vi "DB - OFFSET FETCH.vi"(5 "Include Inactive":bool=TRUE, 6 "OFFSET ROW":i32, 7 "subVI":bool=TRUE, 8 "error in (no error)":errorcluster, 9 "Column to Order BY":string="orderid", 10 "DB.dbo.Table":string="MyDB1.dbo.PartsDetails", 11 "Refnum in":T3) -> (0 "error out":errorcluster, 2 "Data":string[](array[string]), 3 "Refnum out":T3)   [LabVIEW 2013]
uses:
  <vilib>/addons/database/Connection.llb/Conn ObjectReference.ctl
  Controls/DB - DB.Schema.Table.ctl
  <vilib>/addons/database/Connection.llb/Conn Execute.vi
  <vilib>/addons/database/Recordset.llb/Rec Fetch Recordset Data (R).vi
  <vilib>/addons/database/Recordset.llb/Rec Destroy - Connection.vi
  <vilib>/addons/database/Connection.llb/DB Tools Open Connec (String).vi
  <vilib>/addons/database/_DB Variant To Data/Database Variant To Data.xnode
  <vilib>/addons/database/NI_Database_API.lvlib
panel:
  out "DB.Schema.Table":T1
  out "call chain":string[](array[string])
  out "data":string[][](array[string])
  out "QUERY STRING":string
  in  "Connection Information":T2={"Connection "="SQL Server 32bit HPEnvy", "Username"="admin", "Password"="admin123"}
  # "Orders\nPartsDetails\nTransactions"
  # "select * from MyDB1.dbo.Orders WHERE Inactive <> 'X' OR Inactive IS NULL  \nORDER by OrderNo \nOFFSET 1 ROWS FETCH NEXT 1 ROWS ONLY"
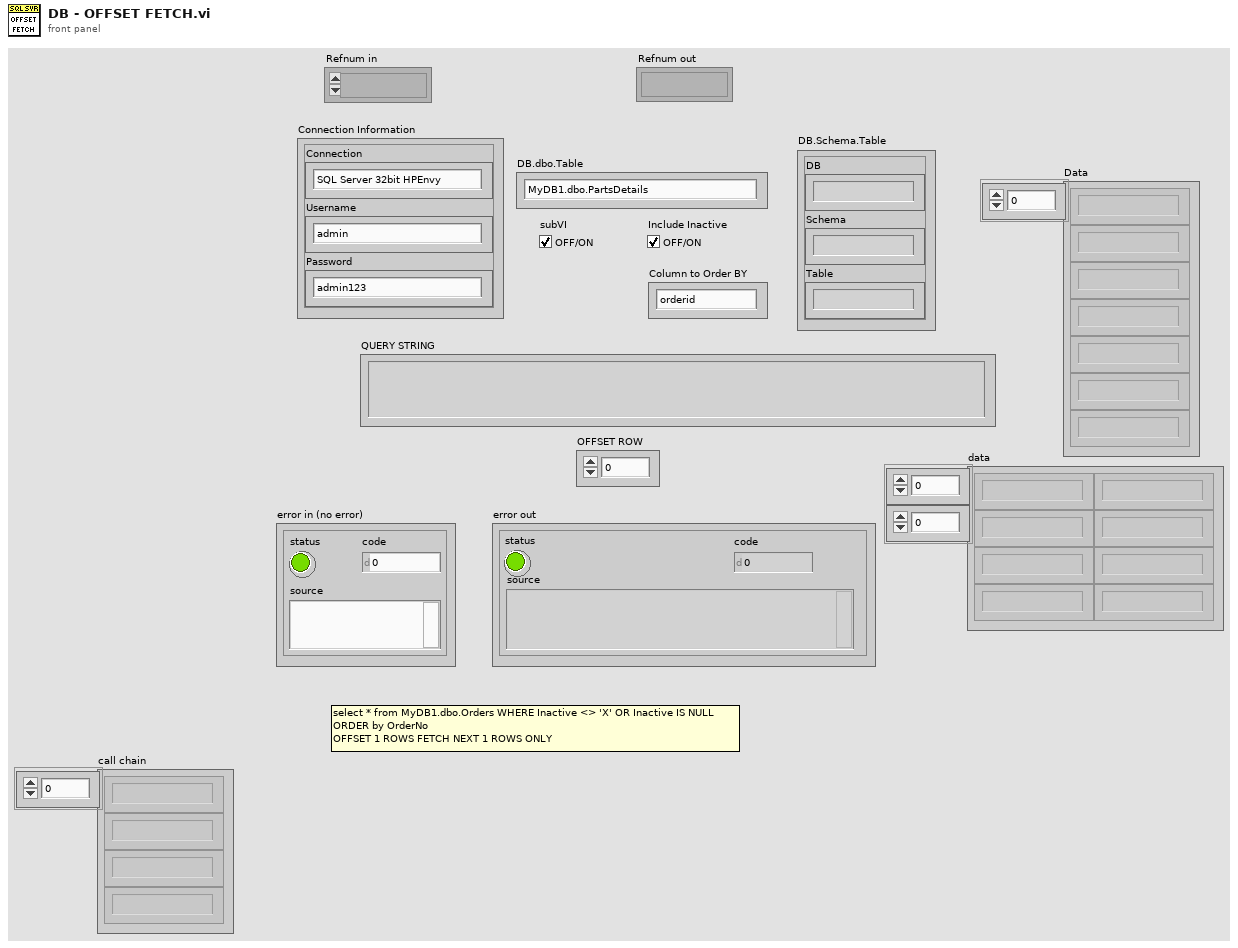
[diagram p1: front panel]
types:
  T1 = typedef "DB - DB.Schema.Table.ctl" = cluster{"DB":string, "Schema":string, "Table":string}
  T2 = cluster{"Connection ":string, "Username":string, "Password":string}
  T3 = typedef "NI_Database_API.lvlib/Conn ObjectReference.ctl" = refnum<k1>
  T4 = typedef "NI_Database_API.lvlib/Rec ObjectReference.ctl" = refnum<k1>
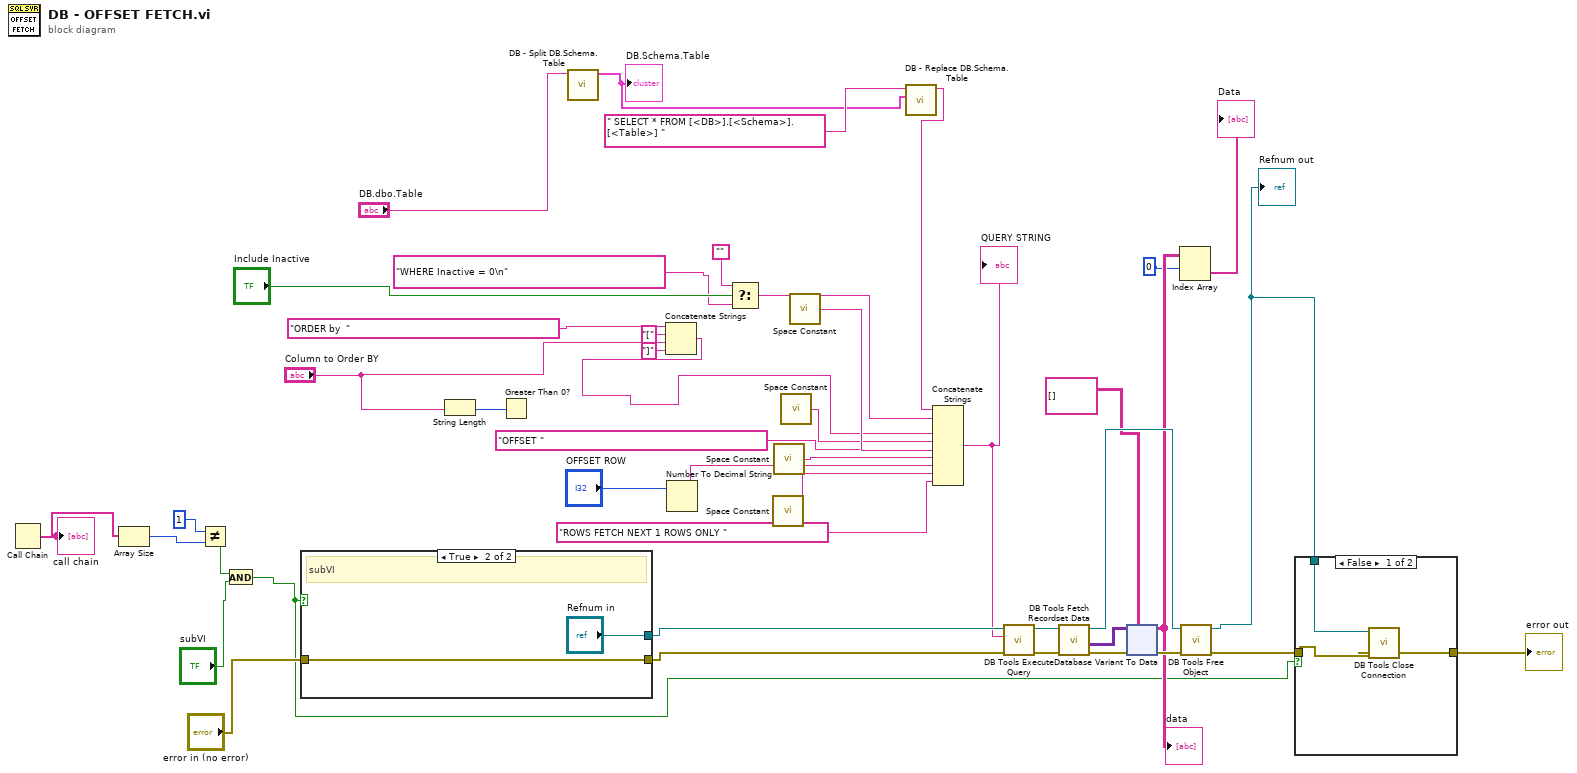
[diagram p0: block diagram]
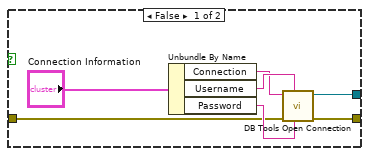
[diagram p3: hidden frame]
diagram:
  n1 = Call Chain() -> (call chain=w20:string[])
  "call chain" <- w20
  n2 = Array Size(array=w20) -> (size(s)=w19:i32)
  n3 = Not Equal?(x=1, y=w19) -> (x != y?=w18:bool)
  n4 = And(x=w18, y="subVI") -> (x .and. y?=w15:bool)
  n5 = case shown="True" w15 {
    tunnel: [w48 "Refnum in"] -> w37
    tunnel: "error in (no error)" -> [w47 w53]
    tunnel: [w46 w53] -> w38
    frame False {
      n6 = Unbundle By Name("Connection Information") -> ("Connection"=w50:string, "Username"=w51:string, "Password"=w49:string)
      n7 = call-poly <vilib>:"DB Tools Open Connection.vi"("password"=w49, "userID"=w51, "error in (no error)"=w47, "connection information"=w50) -> ("error out"=w46:errorcluster, "connection reference"=w48:T3)  [unwired: 4 in]
    }
    frame True {
      # "subVI"
    }
  }
  n8 = String Length(string="Column to Order BY") -> (length=w9:i32)
  n9 = Greater Than 0?(x=w9) -> ()  [unwired: 1 out]
  n10 = call "DB - Split DB.Schema.Table.vi"("DB.Schema.Table"="DB.dbo.Table") -> ("DB.Schema.Table"=w2:T1)  [unwired: 10 in]
  "DB.Schema.Table" <- w2
  n11 = Concatenate Strings("ORDER by  " ("string"), "[" ("string"), "Column to Order BY", "]" ("string")) -> (w7:string)
  n12 = Number To Decimal String(number="OFFSET ROW") -> (decimal integer string=w24:string)  [unwired: 1 in]
  n13 = Select(t="", s="Include Inactive", f="WHERE Inactive = 0\n" ("string")) -> (s? t:f=w10:string)
  n14 = call <vilib>:"Space Constant.vi"() -> ("String"=w23:string)
  n15 = call <vilib>:"Space Constant.vi"() -> ("String"=w26:string)
  n16 = call <vilib>:"Space Constant.vi"() -> ("String"=w27:string)
  n17 = call <vilib>:"Space Constant.vi"() -> ("String"=w28:string)
  n18 = call "DB - Replace DB.Schema.Table.vi"("DB.Schema.Table"=w2, "string in"=" SELECT * FROM [<DB>].[<Schema>].[<Table>] " ("string")) -> ("string out"=w1:string)  [unwired: 8 in, 1 out]
  n19 = Concatenate Strings(w1, w10, w28, w7, w27, "OFFSET " ("string"), w26, w24, w23, "ROWS FETCH NEXT 1 ROWS ONLY " ("string")) -> (w34:string)
  "QUERY STRING" <- w34
  n20 = call-poly <vilib>:"DB Tools Execute Query.vi"("error in (no error)"=w38, "SQL query"=w34, "connection reference"=w37) -> ("error out"=w42:errorcluster, "recordset reference"=w40:T4)  [unwired: 5 in]
  n21 = call-poly <vilib>:"DB Tools Fetch Recordset Data.vi"("error in (no error)"=w42, "recordset reference"=w40) -> ("error out"=w44:errorcluster, "recordset data"=w43:variant[][], "recordset reference out"=w41:T4)  [unwired: 3 in]
  n22 = xnode "Database Variant To Data"("database variant"=w43, "error in (no error)"=w44, "type"=string[][] []) -> ("data"=w35:string[][], "error out"=w45:errorcluster)
  "data" <- w35
  n23 = Index Array(array=w35, index (row)=0 ("disabled index (row)")) -> (element=→"Data":string[])  [unwired: 1 in]
  n24 = call-poly <vilib>:"DB Tools Free Object.vi"("error in (no error)"=w45, "recordset reference"=w41) -> ("error out"=w33:errorcluster, "connection reference"=w31:T3)  [unwired: 8 in]
  "Refnum out" <- w31
  n25 = case shown="False" w15 {
    tunnel: w31 -> [w57 _]
    tunnel: w33 -> [w56 w58]
    tunnel: [w55 w58] -> w36
    frame False {
      n26 = call <vilib>:"DB Tools Close Connection.vi"("error in (no error)"=w56, "connection reference"=w57) -> ("error out"=w55:errorcluster)  [unwired: 5 in]
    }
    frame True {
      # "subVI"
    }
  }
  "error out" <- w36
